vi "si_write_temperature.vi"(9 "INPUT TEMPERATURE":dbl=25.0) -> ()   [LabVIEW 2011]
doc: "This VI sets the the thermal head at any temperature between -15 and 110 degree celsius through the controller.\n\nInputs:\n1. Write Temperature : The required temperature for the thermal head."
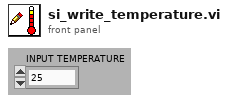
[diagram p1: front panel]
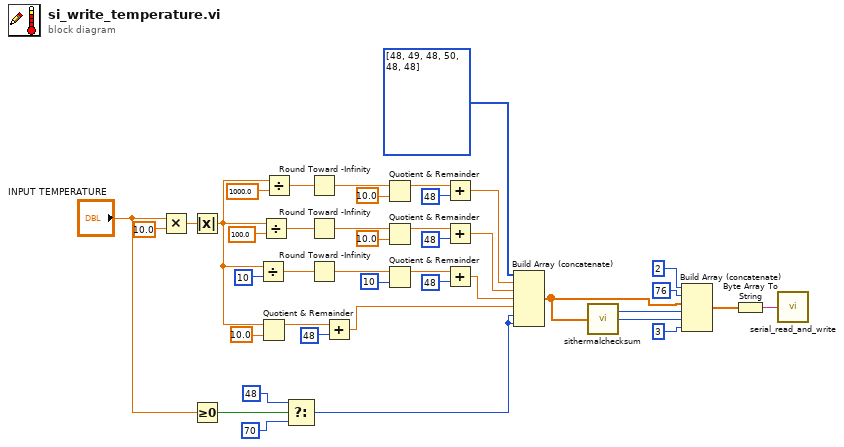
[diagram p0: block diagram]
diagram:
  n1 = Multiply(x="INPUT TEMPERATURE", y=10.0) -> (x*y=w42:dbl)
  n2 = Absolute Value(x=w42) -> (abs(x)=w27:dbl)
  n3 = Greater Or Equal To 0?(x="INPUT TEMPERATURE") -> (x >= 0?=w4:bool)
  n4 = Divide(x=w27, y=i16 10) -> (x/y=w30:dbl)
  n5 = Quotient & Remainder(x=w27, y=10.0) -> (x-y*floor(x/y)=w18:dbl)  [unwired: 1 out]
  n6 = Divide(x=w27, y=100.0) -> (x/y=w34:dbl)
  n7 = Divide(x=w27, y=1000.0) -> (x/y=w38:dbl)
  n8 = Select(t=48, s=w4, f=70) -> (s? t:f=w1:i32)
  n9 = Round Toward -Infinity(1:w38) -> (0:w37:dbl)
  n10 = Round Toward -Infinity(1:w34) -> (0:w33:dbl)
  n11 = Round Toward -Infinity(1:w30) -> (0:w29:dbl)
  n12 = Add(x=w18, y=i16 48) -> (x+y=w14:dbl)
  n13 = Quotient & Remainder(x=w37, y=10.0) -> (x-y*floor(x/y)=w21:dbl)  [unwired: 1 out]
  n14 = Quotient & Remainder(x=w33, y=10.0) -> (x-y*floor(x/y)=w20:dbl)  [unwired: 1 out]
  n15 = Quotient & Remainder(x=w29, y=i16 10) -> (x-y*floor(x/y)=w19:dbl)  [unwired: 1 out]
  n16 = Add(x=w21, y=i16 48) -> (x+y=w17:dbl)
  n17 = Add(x=w20, y=i16 48) -> (x+y=w16:dbl)
  n18 = Add(x=w19, y=i16 48) -> (x+y=w15:dbl)
  n19 = Build Array (concatenate)(i16[] [48, 49, 48, 50, 48, 48] ("Array"), w17, w16, w15, w14, w1, w1) -> (w8:dbl[])
  n20 = call "sithermalchecksum.vi"("Array"=w8) -> ("Lower Checksum"=w6:u8, "Upper Checksum"=w7:u8)
  n21 = Build Array (concatenate)(2, 76, w8, w7, w6, 3) -> (w5:dbl[])
  n22 = Byte Array To String(unsigned byte array=w5) -> (string=w12:string)
  n23 = call "serial_read_and_write.vi"("write buffer"=w12) -> ()  [unwired: 1 in, 1 out]
